vi "J1939 - Workspace Control.vi"() -> ()   [LabVIEW 2015, in "J1939 Workspace Object.lvlib"]
doc: "Sample numeric display item."
uses:
  J1939 Workspace Object.lvlib
  <vilib>/NI Veristand/Display Template Support/Display Template Support.llb/cluster_Screen Item Settings.ctl
  <vilib>/NI Veristand/Display Template Support/Display Template Support.llb/cluster_Graph Scale Settings.ctl
  <vilib>/NI Veristand/Display Template Support/Display Template Support.llb/cluster_Graph Plot Settings.ctl
  Shared/Types/Private Data.ctl
  NationalInstruments.VeriStand.SystemStorage
  <vilib>/NI Veristand/Display Template Support/Display Template Support.llb/enum_Display Template Handler Minimal To Widget Msg.ctl
  <vilib>/NI Veristand/Display Template Support/Display Template Support.llb/enum_Display Template Handler Minimal To Workspace.ctl
  Shared/Types/Error Cluster.ctl
  Shared/Types/Error Types.ctl
  Shared/J1939 Utilities/SubVIs/Convert CAN Arb ID to J1939 ID.vi
  <vilib>/NI Veristand/Display Template Support/Display Template Support.llb/sub_Display Template Handler Custom.vi
  Shared/J1939 Addon Shared.lvlib
  Shared/J1939 Utilities/J1939 Utilities.lvlib
panel:
  out "Device":string
  in  "Errors":bool
  in  "Tab Control":enum32{"DTCs", "Custom RQST", "RAW FRAME"}(tab)
  in  "Refresh Continuous":bool
  in  "Clear DTC":bool
  in  "Refresh DTCs":bool
  in  "DTCs":i32(listbox)
  in  "Addresses":string(tree)
  in  "Refresh Addresses":bool
  out "Response":string
  in  "Request":bool
  in  "PGN":u32
  in  "DA":u8(ring)
  in  "Clear Array":bool
  in  "RAW":bool
  out "Priority":u8 format="%02x"
  out "SA":u8 format="%02x"
  out "PGN":u32 format="%06x"
  in  "Identifier":u32 format="%08x"
  in  "Data":u8[](array[numeric])=[0, 0, 0, 0, 0, 0, 0, 0]
  in  "NIVS.System Definition Root":refnum<k24>
  in  "Cluster":T1={"PGN"=65226, "DA"=0, "CD Path"="", "CD IP"=""}
  in  "Item.Data":T2
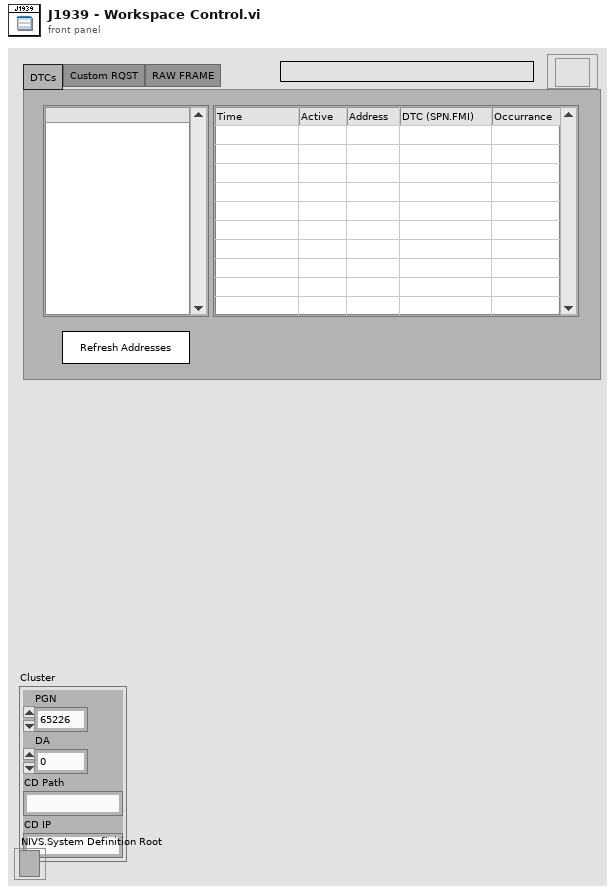
[diagram p1: front panel]
types:
  T1 = typedef "J1939 Addon Shared.lvlib/Private Data.ctl" = cluster{"PGN":u32, "DA":u8, "CD Path":string, "CD IP":string}
  T2 = typedef "cluster_Screen Item Settings.ctl" = cluster{"Template VI":string, "Position X":i32, "Position Y":i32, "Custom":string, "Show Title Bar":bool, "ID":i32, "Always On Top":bool, "Allow Resize":bool, "Allow Minimize":bool, "Allow Close":bool, "Size to Screen":bool, "Screen.ID":i32, "State":enum16{"Normal", "New"}, "Title":string, "Window Bounds":cluster{"[0]":i16, "[1]":i16, "[2]":i16, "[3]":i16}, "Channel Ref":u64, "Unit":string, "Default Units?":bool, "Flash Limit?":bool, "Color 1":u32, "Color 2":u32, "Color 3":u32, "Color 4":u32, "Bck Color":u32, "Fore Color":u32, "Limit 1":dbl, "Limit 2":dbl, "Limit 3":dbl, "Limit 4":dbl, "Limit Mode 1":i32, "Limit Mode 2":i32, "Limit Mode 3":i32, "Limit Mode 4":i32, "Scale Precision":i32, "Scale Min":dbl, "Scale Max":dbl, "Format":i32, "Precision":i32, "Background Type":i32, "IDs":i32[], "Units":string[], "Labels":string[], "Scale Factor":dbl, "Scale Offset":dbl, "YScale Index":u32[], "XScale":T3, "YScales":T3[], "Plots":T4[], "Update Period":dbl, "History Length":dbl, "My.Ref":refnum<vi>, "Is Control?":bool, "Channel Paths":string[], "Custom Data":variant}
  T3 = typedef "cluster_Graph Scale Settings.ctl" = cluster{"Format":u8, "Precision":u8, "Fit":u8, "Label":string, "Use Default Label":bool, "Label Visible":bool, "Min":dbl, "Max":dbl}
  T4 = typedef "cluster_Graph Plot Settings.ctl" = cluster{"Bar Style":u8, "Fill To":i16, "Fill/PtColor":u32, "Line Style":u8, "Line Width":u8, "Color":u32, "Interp":u8, "Point Style":u8}
  T5 = typedef "enum_Display Template Handler Minimal To Workspace.ctl" = cluster{"Operation":enum16{"SetCustomData", "DeleteItem"}, "Data":variant}
  T6 = typedef "enum_Display Template Handler Minimal To Widget Msg.ctl" = enum16{"Stop", "LaunchConfigDialog"}
  T7 = typedef "J1939 Addon Shared.lvlib/Error Cluster.ctl" = cluster{"error out":errorcluster, "Enum":T8, "Address":u8, "Timestamp":timestamp}
  T8 = typedef "J1939 Addon Shared.lvlib/Error Types.ctl" = enum16{"Request", "RAW Generation", "Clear Active DTCs", "Clear Previous DTCs", "Addresses", "TLAs", "Get Active DTCs", "Get Previous DTCs"}
  T9 = typedef "NI STM.lvlib/TCP Connection Info.ctl" = cluster{"connection ID":refnum<k5>, "meta data":T10[]}
  T10 = typedef "NI STM.lvlib/MetaDataElement.ctl" = string
  T11 = enum8{"Enabled", "Disabled", "Disabled and Grayed Out"}
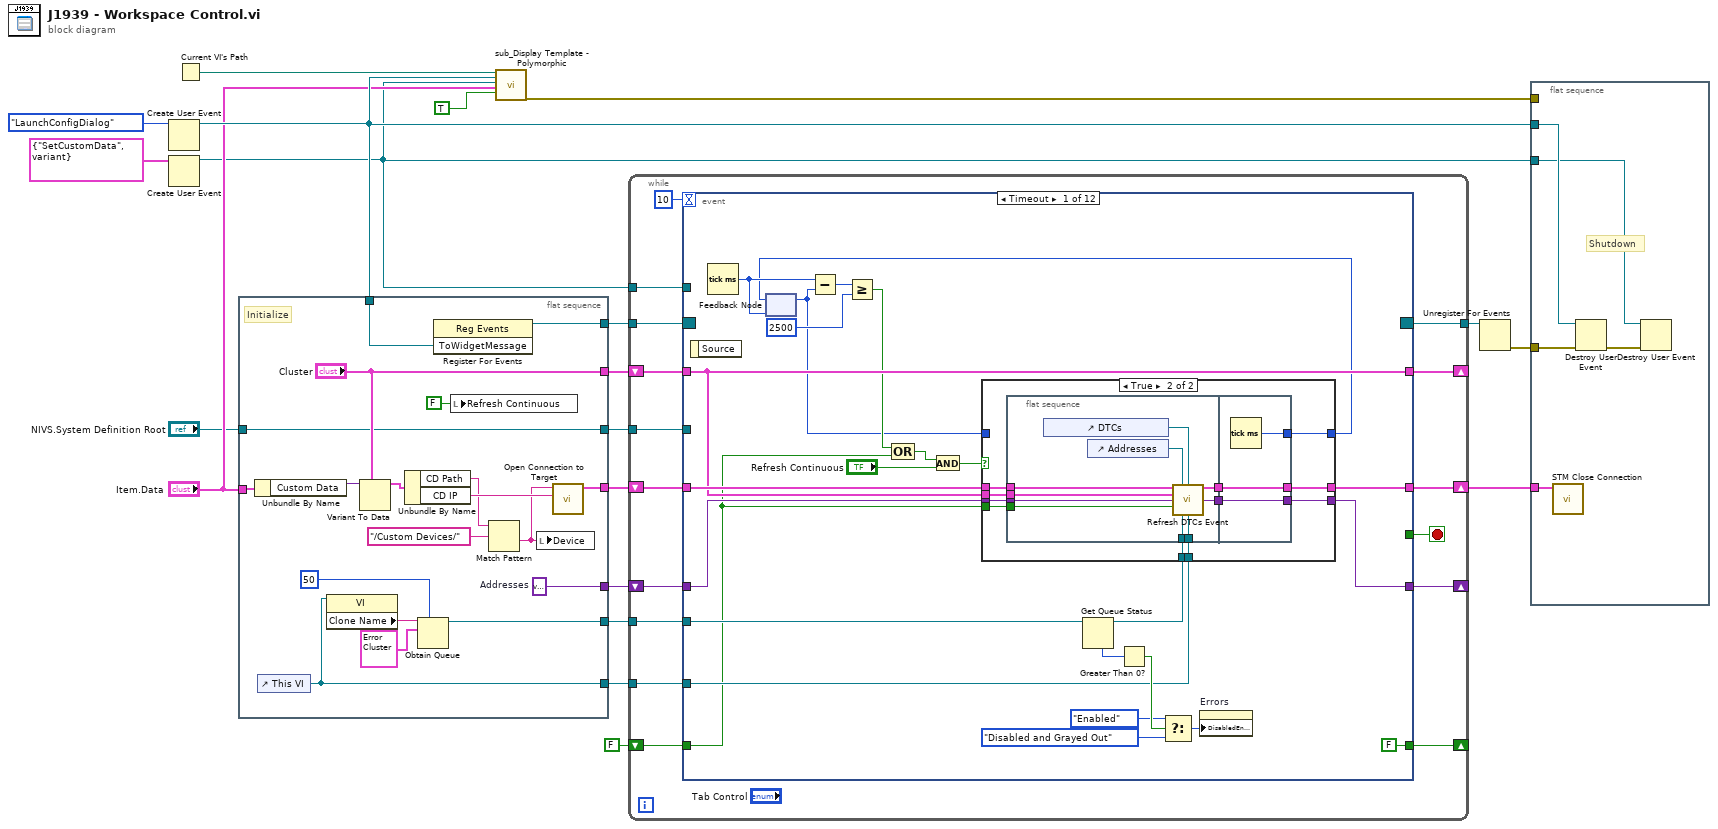
[diagram p0: block diagram]
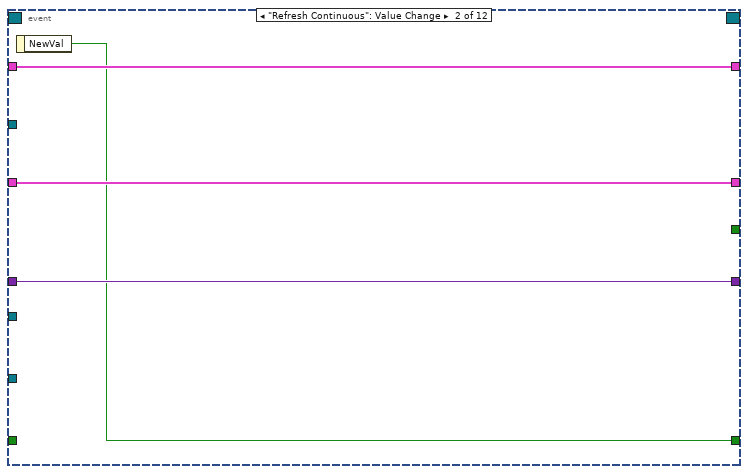
[diagram p3: hidden frame]
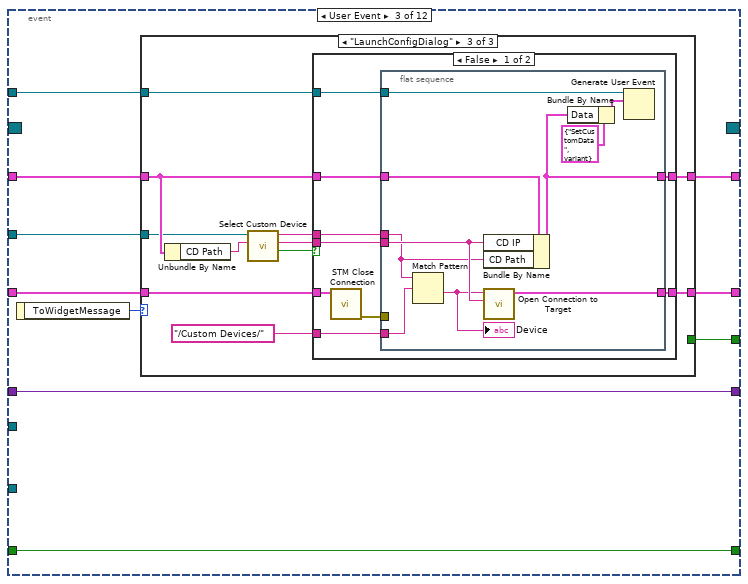
[diagram p4: hidden frame]
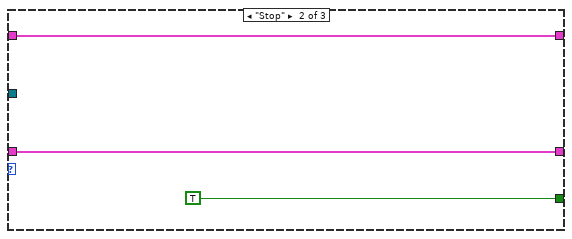
[diagram p6: hidden frame]
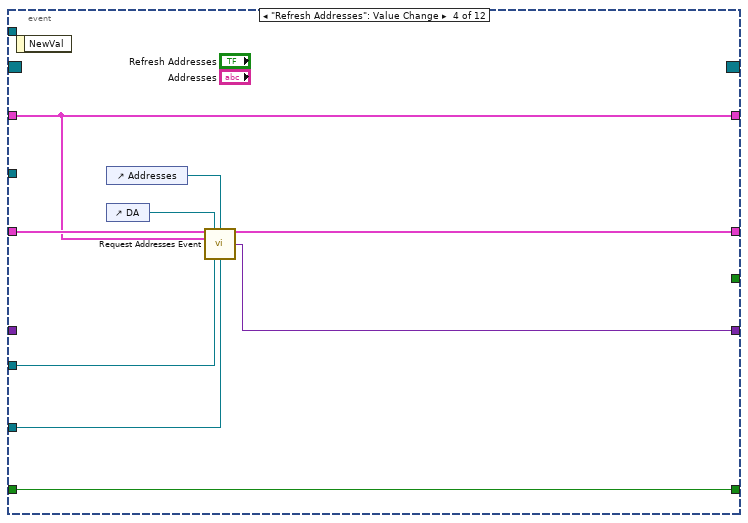
[diagram p8: hidden frame]
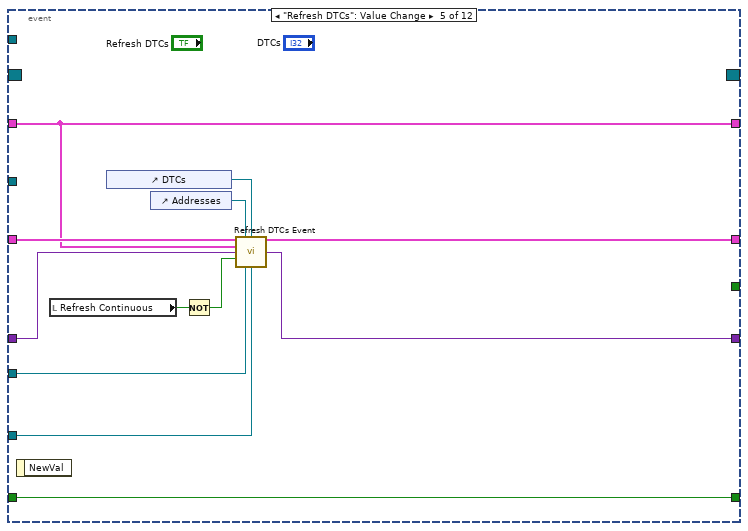
[diagram p9: hidden frame]
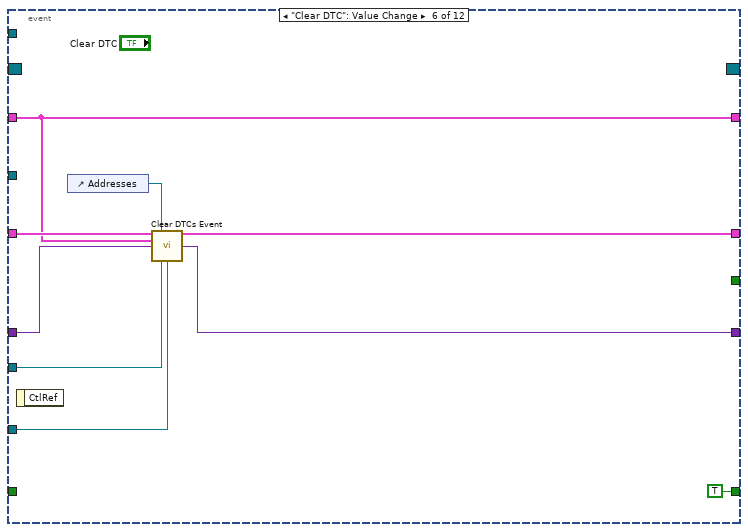
[diagram p10: hidden frame]
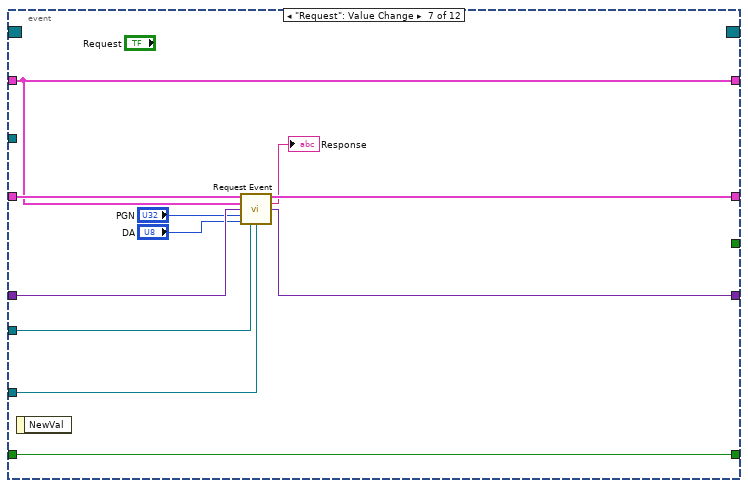
[diagram p11: hidden frame]
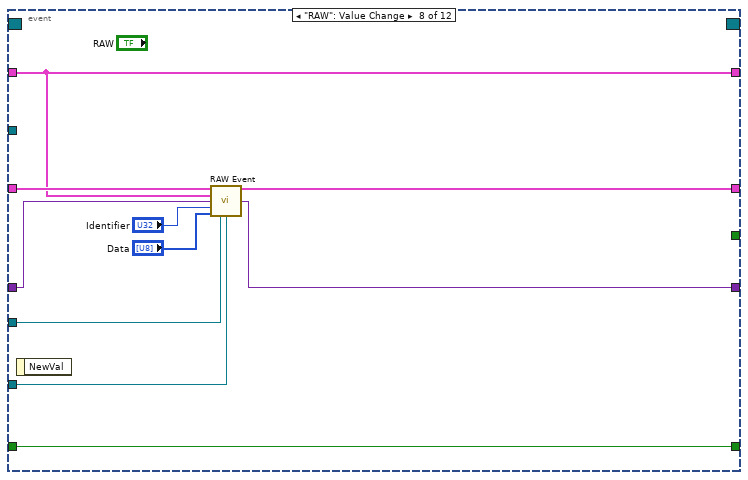
[diagram p12: hidden frame]
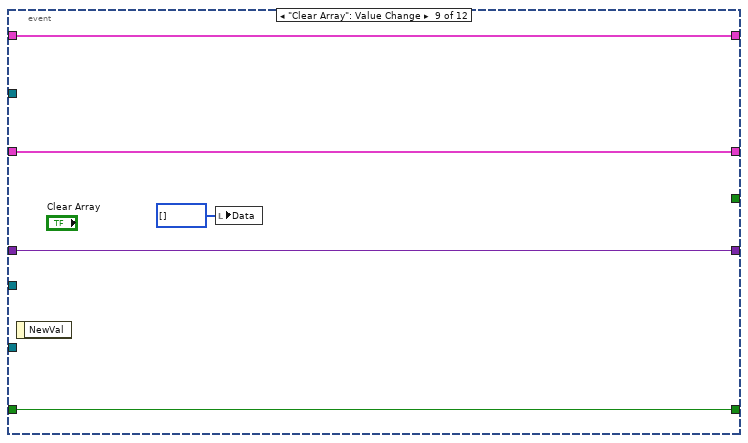
[diagram p13: hidden frame]
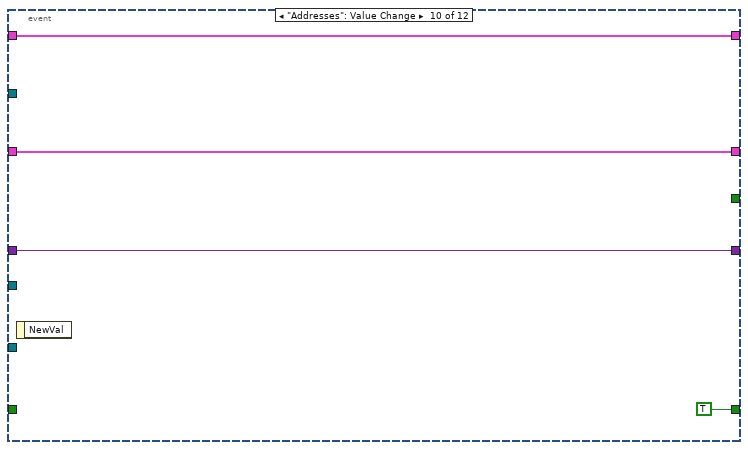
[diagram p14: hidden frame]
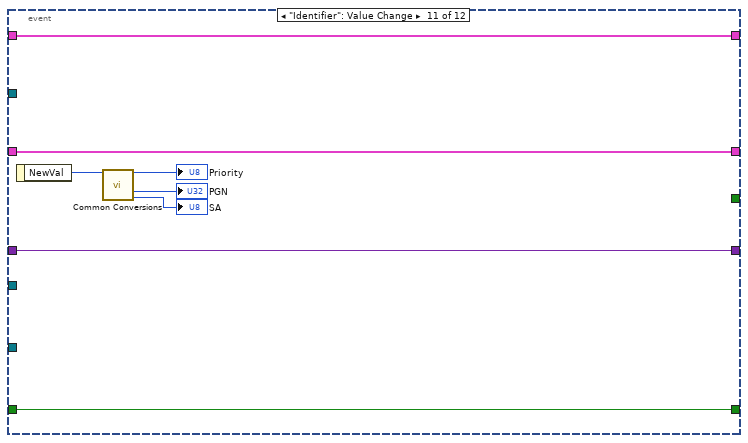
[diagram p15: hidden frame]
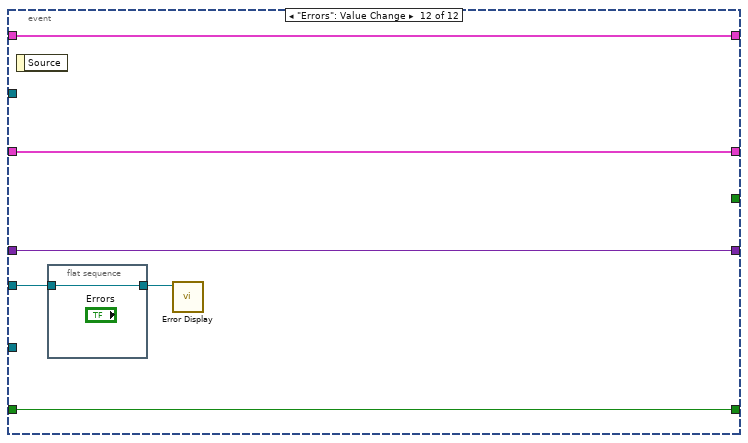
[diagram p16: hidden frame]
diagram:
  n1 = Create User Event(user event datatype=enum_Display_Template_Handler_Minimal_To_Widget_Msg."LaunchConfigDialog" ("ToWidgetMessage")) -> (user event=w15:refnum<user-event>)  [unwired: 1 in, 1 out]
  n2 = Create User Event(user event datatype=T5 {"Operation"=enum."SetCustomData", "Data"=variant} ("Data")) -> (user event=w11:refnum<user-event>)  [unwired: 1 in, 1 out]
  n3 = Current VI's Path() -> (path=w13:path)
  n4 = flat-sequence {
    tunnel: [w39] -> w18
    tunnel: w15 -> [w38]
    tunnel: "Item.Data" -> [w37]
    tunnel: ["Cluster"] -> w9
    tunnel: [w26] -> w8
    tunnel: [w32] -> w6
    tunnel: [w33] -> w5
    tunnel: "NIVS.System Definition Root" -> [w32]
    tunnel: [w30] -> w3
    tunnel: [w22] -> w2
    frame #0 {
      w33 = variant  # Addresses
      # "Initialize"
      n5 = Unbundle By Name(w37) -> ("Custom Data"=w36:variant)
      n6 = control-ref of="This VI"() -> (w22:refnum<vi>)
      n7 = property class="VI"(reference=w22) -> ("Clone Name"=w31:string)  [unwired: 1 in, 2 out]
      n8 = Variant To Data(type="Cluster", Variant=w36) -> (data=w35:T1)  [unwired: 1 in, 1 out]
      n9 = Unbundle By Name(w35) -> ("CD Path"=w24:string, "CD IP"=w27:string)
      n10 = Obtain Queue(max queue size (-1, unlimited)=50, name (unnamed)=w31, element data type=T7 {"error out"={"status"=FALSE, "code"=0, "source"=""}, "Enum"=enum."Request", "Address"=0, "Timestamp"=timestamp(0 s since 1904-01-01)} ("Error Cluster")) -> (queue out=w30:refnum<queue>)  [unwired: 2 in, 2 out]
      n11 = register-events(w38) -> (reference out=w39:refnum<event-registration>)  [unwired: 2 in, 1 out]
      n12 = local write "Refresh Continuous"(FALSE ("Refresh Continuous")) -> ()
      n13 = Match Pattern(string=w24, regular expression="/Custom Devices/") -> (after substring=w23:string)  [unwired: 1 in, 3 out]
      n14 = local write "Device"(w23) -> ()
      n15 = call "Open Connection to Target.vi"("IP Address"=w27, "TCP Service"=w23) -> ("connection info"=w26:T9)  [unwired: 8 in, 1 out]
    }
  }
  n16 = call-poly <vilib>:"sub_Display Template - Polymorphic.vi"("Parent.Path"=w13, "ToWidgetEvent"=w15, "ToWorkspace"=w11, "Item.Data"="Item.Data", "Resizable"=TRUE) -> ("error out"=w20:errorcluster)  [unwired: 1 in, 13 out]
  n17 = while {
    tunnel: w18 -> [w55]
    tunnel: [w53] -> w17
    tunnel: w11 -> [w52]
    shift-right: [w50] -> _
    shift-left: w9 -> [w51]
    shift-right: [w48] -> w7
    shift-left: w8 -> [w49]
    tunnel: w6 -> [w47]
    shift-right: [w46] -> _
    shift-left: w5 -> [w45]
    tunnel: w3 -> [w44]
    tunnel: w2 -> [w42]
    shift-right: [w41] -> _
    shift-left: FALSE -> [w40]
    stop <- w54 stop-if-true
    n18 = event shown="[0] Timeout" {
      selector: w55 -> [_ _ _ _ _ _ _ _ _ _ _ _]
      dyn-events: [_ _ _ _ _ _ _ _ _ _ _ _] -> w53
      timeout: 10 -> [_ _ _ _ _ _ _ _ _ _ _ _]
      tunnel: [_ _ w119 _ _ _ _ _ _ _ _ _] -> w54
      tunnel: w52 -> [_ _ w118 _ _ _ _ _ _ _ _ _]
      tunnel: w51 -> [w69 w108 w112 w165 w174 w182 w193 w203 w211 w215 w225 w229]
      tunnel: [w69 w108 w117 w165 w174 w182 w193 w203 w211 w215 w225 w229] -> w50
      tunnel: w49 -> [w71 w109 w116 w166 w178 w187 w198 w208 w212 w216 w224 w231]
      tunnel: [w70 w109 w115 w164 w175 w186 w197 w207 w212 w216 w224 w231] -> w48
      tunnel: w47 -> [_ _ w114 _ _ _ _ _ _ _ _ _]
      tunnel: [w72 w110 w113 w163 w176 w184 w194 w206 w213 w217 w223 w230] -> w46
      tunnel: w45 -> [w73 w110 w113 _ w177 w185 w195 w205 w213 w217 w223 w230]
      tunnel: w44 -> [w79 _ _ w162 w173 w183 w196 w204 _ _ _ w227]
      tunnel: w42 -> [w61 _ _ w161 w172 w181 w192 w202 _ _ _ _]
      tunnel: [FALSE w107 w111 w158 w169 TRUE w188 w199 w209 TRUE w218 w226] -> w41
      tunnel: w40 -> [w58 _ w111 w158 w169 _ w188 w199 w209 _ w218 w226]
      event Timeout {
        n19 = event-data() -> ()  [unwired: 2 out]
        n20 = Tick Count (ms)() -> (millisecond timer value=w66:u32)
        n21 = feedback #1(w66) -> (w56:u32)
        n22 = Subtract(x=w66, y=w56) -> (x-y=w68:u32)
        n23 = Greater Or Equal?(x=w68, y=u32 2500) -> (x >= y?=w65:bool)
        n24 = Compound Arithmetic op=OR(w65, w58) -> (w59:bool)
        n25 = And(x=w59, y="Refresh Continuous") -> (x .and. y?=w63:bool)
        n26 = Get Queue Status(queue=w79) -> (queue out=w62:refnum<queue>, # elements in queue=w78:i32)  [unwired: 2 in, 6 out]
        n27 = case shown="True" w63 {
          tunnel: w73 -> [w82 w93]
          tunnel: [w82 w92] -> w72
          tunnel: w71 -> [w81 w91]
          tunnel: [w81 w90] -> w70
          tunnel: w69 -> [_ w89]
          tunnel: w62 -> [_ w88]
          tunnel: w61 -> [_ w87]
          tunnel: w58 -> [_ w86]
          tunnel: [w80 w83] -> w57
          tunnel: w56 -> [w80 _]
          frame False {
          }
          frame True {
            n28 = flat-sequence {
              tunnel: w93 -> [w101]
              tunnel: w91 -> [w99]
              tunnel: w89 -> [w97]
              tunnel: w88 -> [w96]
              tunnel: w87 -> [w95]
              tunnel: w86 -> [w94]
              tunnel: [w100] -> w85
              tunnel: [w98] -> w84
              tunnel: [w105] -> w90
              tunnel: [w106] -> w92
              tunnel: w85 -> [w106]
              tunnel: w84 -> [w105]
              tunnel: [w104] -> w83
              frame #0 {
                n29 = control-ref of="DTCs"() -> (w102:refnum<vi>)
                n30 = control-ref of="Addresses"() -> (w103:refnum<vi>)
                n31 = call "Refresh DTCs Event.vi"("connection info"=w99, "Addresses"=w103, "DTCs"=w102, "State Variables"=w97, "Address Lookup Table"=w101, "To Top (T)"=w94, "Error Q"=w96, "VI Ref"=w95) -> ("connection info"=w98:T9, "Address Lookup Table Out"=w100:variant)  [unwired: 6 in]
              }
              frame #1 {
                n32 = Tick Count (ms)() -> (millisecond timer value=w104:u32)
              }
            }
          }
        }
        n33 = feedback-in #1(w57) -> ()
        n34 = Greater Than 0?(x=w78) -> (x > 0?=w77:bool)
        n35 = Select(t=T11."Enabled" ("Disabled"), s=w77, f=T11."Disabled and Grayed Out") -> (s? t:f=w74:T11)
        n36 = property on="Errors" class="Bool"("DisabledEnum"=w74) -> ()  [unwired: 2 in, 2 out]
      }
      event "Refresh Continuous": Value Change {
        n37 = event-data() -> ("NewVal"=w107:bool)  [unwired: 1 out]
      }
      event User Event {
        n38 = event-data() -> ("ToWidgetMessage"=w120:T6)  [unwired: 1 out]
        n39 = case shown="\"LaunchConfigDialog\"" w120 {
          tunnel: [_ TRUE _] -> w119
          tunnel: w118 -> [_ _ w136]
          tunnel: w112 -> [w122 w124 w135]
          tunnel: [w122 w124 w132] -> w117
          tunnel: w116 -> [w121 w123 w126]
          tunnel: [w121 w123 w134] -> w115
          tunnel: w114 -> [_ _ w133]
          frame Default {
          }
          frame "Stop" {
          }
          frame "LaunchConfigDialog" {
            n40 = Unbundle By Name(w135) -> ("CD Path"=w130:string)
            n41 = call "Select Custom Device.vi"("CD Path"=w130, "NIVS.System Definition Root"=w133) -> ("Cancelled?"=w127:bool, "IP Address"=w131:string, "Custom Device Path Out"=w128:string)  [unwired: 7 in]
            n42 = case shown="False" w127 {
              tunnel: w136 -> [w145 _]
              tunnel: w135 -> [w144 w157]
              tunnel: [w143 w156] -> w134
              tunnel: [w142 w157] -> w132
              tunnel: w131 -> [w141 _]
              tunnel: "/Custom Devices/" ("regular expression") -> [w140 _]
              tunnel: w128 -> [w139 _]
              tunnel: w126 -> [w138 w156]
              frame False {
                n43 = call "STM Close Connection.vi"("connection info"=w138) -> ("error out"=w137:errorcluster)  [unwired: 10 in]
                n44 = flat-sequence {
                  tunnel: w145 -> [w155]
                  tunnel: w144 -> [w154]
                  tunnel: [w153] -> w143
                  tunnel: [w152] -> w142
                  tunnel: w141 -> [w151]
                  tunnel: w140 -> [w147]
                  tunnel: w139 -> [w146]
                  tunnel: w137 -> [_]
                  frame #0 {
                    n45 = Match Pattern(string=w146, regular expression=w147) -> (after substring=w150:string)  [unwired: 1 in, 3 out]
                    "Device" <- w150
                    n46 = Bundle By Name(cluster=w154, "CD IP"=w151, "CD Path"=w146) -> (w152:T1)
                    n47 = call "Open Connection to Target.vi"("IP Address"=w151, "TCP Service"=w150) -> ("connection info"=w153:T9)  [unwired: 8 in, 1 out]
                    n48 = Bundle By Name(cluster=T5 {"Operation"=enum."SetCustomData", "Data"=variant} ("event data"), "Data"=w152) -> (w148:T5)
                    n49 = Generate User Event(user event=w155, event data cluster=w148) -> ()  [unwired: 2 in, 2 out]
                  }
                }
              }
              frame True {
              }
            }
          }
        }
      }
      event "Refresh Addresses": Value Change {
        n50 = event-data() -> ()  [unwired: 2 out]
        n51 = control-ref of="Addresses"() -> (w159:refnum<vi>)
        n52 = control-ref of="DA"() -> (w160:refnum<vi>)
        n53 = call "Request Addresses Event.vi"("connection info"=w166, "DA"=w160, "Addresses"=w159, "State Variables"=w165, "Error Q"=w162, "VI Ref"=w161) -> ("connection info"=w164:T9, "Address Lookup Table Out"=w163:variant)  [unwired: 8 in]
      }
      event "Refresh DTCs": Value Change {
        n54 = event-data() -> ()  [unwired: 2 out]
        n55 = local read "Refresh Continuous"() -> (w168:bool)
        n56 = control-ref of="DTCs"() -> (w170:refnum<vi>)
        n57 = control-ref of="Addresses"() -> (w171:refnum<vi>)
        n58 = Not(x=w168) -> (.not. x?=w167:bool)
        n59 = call "Refresh DTCs Event.vi"("connection info"=w178, "Addresses"=w171, "DTCs"=w170, "State Variables"=w174, "Address Lookup Table"=w177, "To Top (T)"=w167, "Error Q"=w173, "VI Ref"=w172) -> ("connection info"=w175:T9, "Address Lookup Table Out"=w176:variant)  [unwired: 6 in]
      }
      event "Clear DTC": Value Change {
        n60 = event-data() -> ()  [unwired: 2 out]
        n61 = control-ref of="Addresses"() -> (w180:refnum<vi>)
        n62 = call "Clear DTCs Event.vi"("connection info"=w187, "Addresses"=w180, "State Variables"=w182, "Address Lookup Table"=w185, "Error Q"=w183, "VI Ref"=w181) -> ("connection info"=w186:T9, "Address Lookup Table Out"=w184:variant)  [unwired: 8 in]
      }
      event "Request": Value Change {
        n63 = event-data() -> ()  [unwired: 2 out]
        n64 = call "Request Event.vi"("connection info"=w198, "State Variables"=w193, "Address Lookup Table"=w195, "PGN"="PGN", "DA"="DA", "Error Q"=w196, "VI Ref"=w192) -> ("connection info"=w197:T9, "Response"=→"Response":string, "Address Lookup Table Out"=w194:variant)  [unwired: 6 in]
      }
      event "RAW": Value Change {
        n65 = event-data() -> ()  [unwired: 2 out]
        n66 = call "RAW Event.vi"("connection info"=w208, "State Variables"=w203, "Address Lookup Table"=w205, "Identifier"="Identifier", "Data"="Data", "Error Q"=w204, "VI Ref"=w202) -> ("connection info"=w207:T9, "Address Lookup Table Out"=w206:variant)  [unwired: 7 in]
      }
      event "Clear Array": Value Change {
        n67 = event-data() -> ()  [unwired: 2 out]
        n68 = local write "Data"(u8[] [] ("Data")) -> ()
      }
      event "Addresses": Value Change {
        n69 = event-data() -> ()  [unwired: 2 out]
      }
      event "Identifier": Value Change {
        n70 = event-data() -> ("NewVal"=w219:u32)  [unwired: 1 out]
        n71 = call-poly "Common Conversions.vi"("Arb ID"=w219) -> ("Priority"=→"Priority":u8, "PGN"=→"PGN":u32, "Source Address"=→"SA":u8)  [unwired: 11 in, 1 out]
      }
      event "Errors": Value Change {
        n72 = event-data() -> ()  [unwired: 2 out]
        n73 = flat-sequence {
          tunnel: [w232] -> w228
          tunnel: w227 -> [w232]
          frame #0 {
          }
        }
        n74 = call "Error Display.vi"("queue out"=w228) -> ()  [unwired: 11 in]
      }
    }
  }
  n75 = Unregister For Events(event registration refnum=w17) -> (error out=w16:errorcluster)  [unwired: 1 in]
  n76 = flat-sequence {
    tunnel: w20 -> [_]
    tunnel: w16 -> [w236]
    tunnel: w15 -> [w237]
    tunnel: w11 -> [w234]
    tunnel: w7 -> [w233]
    frame #0 {
      # "Shutdown"
      n77 = call "STM Close Connection.vi"("connection info"=w233) -> ()  [unwired: 10 in, 1 out]
      n78 = Destroy User Event(user event=w237, error in=w236) -> (error out=w235:errorcluster)
      n79 = Destroy User Event(user event=w234, error in=w235) -> ()  [unwired: 1 out]
    }
  }
